vi "Read Counter Driven Output Module.vi"(8 "error in":errorcluster, 11 "module in":refnum<class "Module.lvclass">) -> (0 "error out":errorcluster, 1 "drive from slot":T1, 2 "channel settings":T2[](array[typedef]), 3 "module out":refnum<class "Module.lvclass">)   [LabVIEW 2017, in "Scan Engine Scripting.lvlib" / "Module.lvclass"]
uses:
  Module.lvclass
  Mode Classes/Controls/counter driven output channel settings.ctl
  Channel Classes/Counter Driven Output Channel/Counter Driven State.ctl
  Mode Classes/Counter Driven Output Mode/Drive from Slot.ctl
  Mode Classes/Counter Driven Output Mode/Counter Driven Output Mode.lvclass
  Channel Classes/Counter Driven Output Channel/Counter Driven Output Channel.lvclass
  Scan Engine Scripting.lvlib
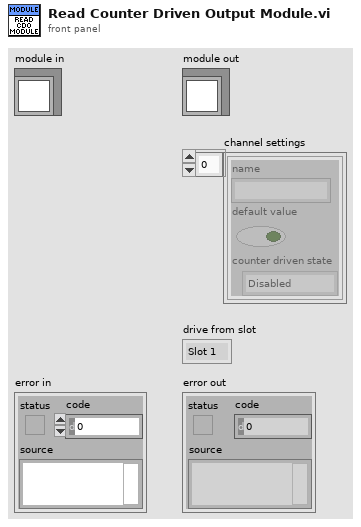
[diagram p1: front panel]
types:
  T1 = typedef "Scan Engine Scripting.lvlib/Counter Driven Output Mode.lvclass/Drive from Slot.ctl" = enum16{"Slot 1", "Slot 2", "Slot 3", "Slot 4", "Slot 5", "Slot 6", "Slot 7", "Slot 8"}
  T2 = typedef "Scan Engine Scripting.lvlib/counter driven output channel settings.ctl" = cluster{"name":string, "default value":bool, "counter driven state":T3}
  T3 = typedef "Scan Engine Scripting.lvlib/Counter Driven Output Channel.lvclass/Counter Driven State.ctl" = enum16{"Disabled", "Enabled"}
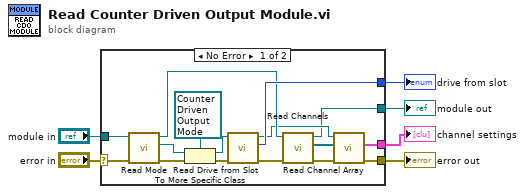
[diagram p0: block diagram]
diagram:
  n1 = case shown="No Error" "error in" {
    selector: "error in" -> [w21 w24]
    tunnel: [w9 w24] -> w3
    tunnel: [w7 w23] -> w4
    tunnel: "module in" -> [w22 w23]
    tunnel: [w15 _] -> w2
    tunnel: [w8 _] -> w1
    frame No Error {
      n2 = call-dynamic "Read Mode.vi"("error in"=w21, "module in"=w22) -> ("error out"=w18:errorcluster, "mode"=w20:refnum<class "Mode.lvclass">, "module out"=w13:refnum<class "Module.lvclass">)  [unwired: 7 in]
      n3 = To More Specific Class(target class=refnum<class "Counter Driven Output Mode.lvclass"> refnum ("Scan Engine Scripting.lvlib:Counter Driven Output Mode.lvclass"), reference=w20, error in=w18) -> (specific class reference=w17:refnum<class "Counter Driven Output Mode.lvclass">, error out=w16:errorcluster)
      n4 = call-dynamic "Read Drive from Slot.vi"("error in"=w16, "counter driven output mode in"=w17) -> ("error out"=w14:errorcluster, "drive from slot"=w15:T1, "counter driven output mode out"=w12:refnum<class "Counter Driven Output Mode.lvclass">)  [unwired: 7 in]
      n5 = call-dynamic "Read Channels.vi"("error in"=w14, "module in"=w13) -> ("error out"=w10:errorcluster, "channels"=w11:refnum<class "Channel.lvclass">[], "module out"=w7:refnum<class "Module.lvclass">)  [unwired: 7 in]
      n6 = call "Read Channel Array.vi"("error in"=w10, "channels"=w11, "counter driven output mode in"=w12) -> ("error out"=w9:errorcluster, "channel settings"=w8:T2[])  [unwired: 6 in, 1 out]
    }
    frame Error {
    }
  }
  "error out" <- w3
  "module out" <- w4
  "channel settings" <- w1
  "drive from slot" <- w2
